vi "Write Current Packet Size.vi"(8 "error in (no error)":errorcluster, 10 "Current Packet Size":i32, 11 "Packet in":refnum<class "Packet.lvclass">) -> (0 "error out":errorcluster, 3 "Packet out":refnum<class "Packet.lvclass">)   [LabVIEW 2013, in "Packet.lvclass"]
uses:
  Packet.lvclass
  Packet.lvclass/Packet.ctl
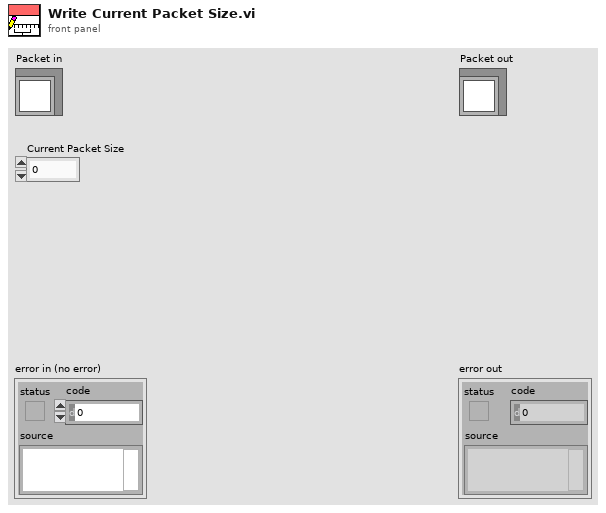
[diagram p1: front panel]
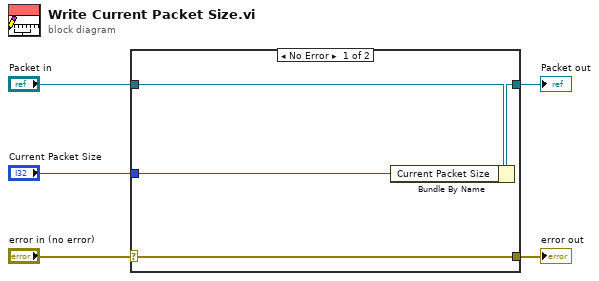
[diagram p0: block diagram]
diagram:
  n1 = case shown="No Error" "error in (no error)" {
    selector: "error in (no error)" -> [w9 w10]
    tunnel: [w9 w10] -> w4
    tunnel: [w7 w11] -> w2
    tunnel: "Packet in" -> [w8 w11]
    tunnel: "Current Packet Size" -> [w6 _]
    frame No Error {
      n2 = Bundle By Name(cluster=w8, "Current Packet Size"=w6) -> (w7:refnum<class "Packet.lvclass">)
    }
    frame Error {
    }
  }
  "error out" <- w4
  "Packet out" <- w2
